vi "RudderToPoint.vi"(0 "Waypoint":T2 {"North" format="%#_10f"; "East" format="%#_8f"}, 1 "Robot Location":T2 {"North" format="%#_10f"; "East" format="%#_8f"}, 2 "Robot Heading":dbl, 3 "Angle to Check":dbl) -> (7 "Suggested Rudder Setpoint":T1 min=-1.0 max=1.0)   [LabVIEW 2012]
doc: "Takes in an angle to check, and returns a goodness value related to how close said angle is to the angle between the robot and the waypoint.\n\n**I find the above statement very unclear. What this vi should do now (perhaps this wasn't the original point, I can't tell) is take in the angle of the boat relative to the target, and use the rudder to point the boat at the target. This is done by putting a control loop around the boat-to-waypoint angle and making it go to zero. The control loop should be adjusted so that you get a more extreme reaction from the rudder at lower speeds. At a very low speed cutoff perhaps the rudder should just be set to 0, to save battery from the rudder twitching back and forth.**\n\nModified by Eric Schneider, Jan. 2014"
uses:
  Data/TypeDefs/UTM Location.ctl
  Data/TypeDefs/Rudder Set Suggestions.ctl
  Utilities/Math/Angles/Angle/Angle.lvclass
panel:
  out "Goodness":dbl
  # "TODO: Update the awful documentation"
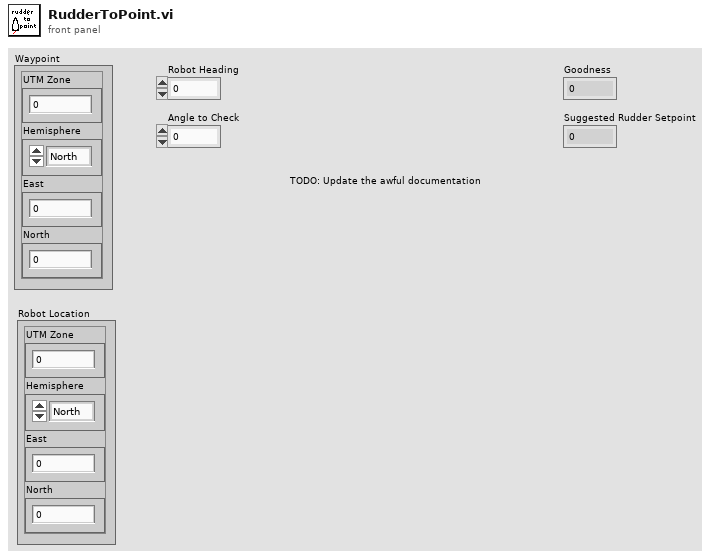
[diagram p1: front panel]
types:
  T1 = typedef "Rudder Set Suggestions.ctl" = dbl
  T2 = typedef "UTM Location.ctl" = cluster{"UTM Zone":dbl, "Hemisphere":enum16{"North", "South"}, "East":dbl, "North":dbl}
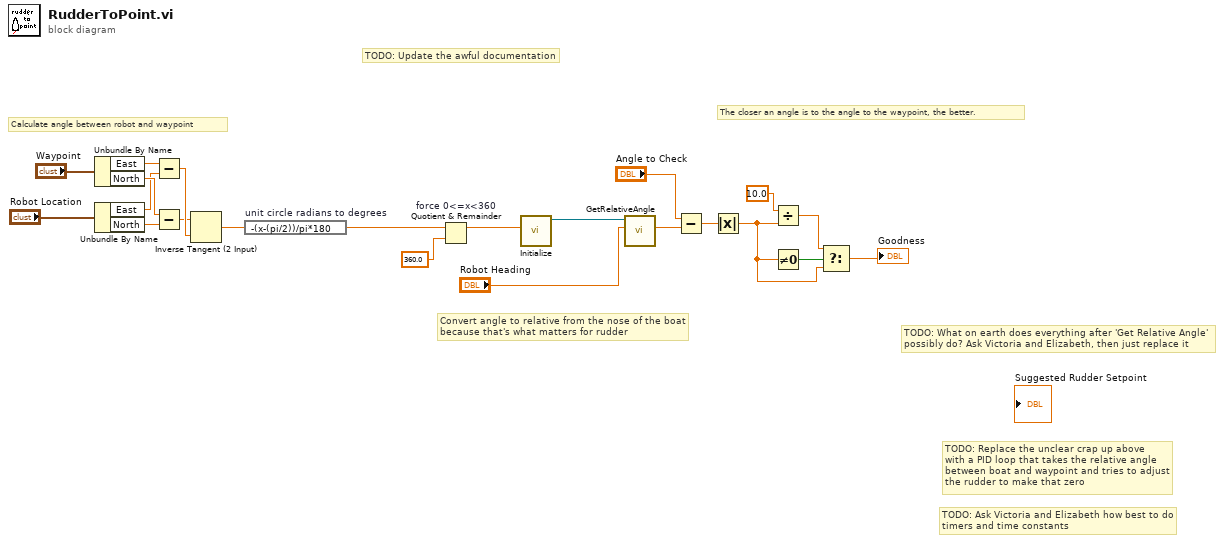
[diagram p0: block diagram]
diagram:
  # "TODO: Ask Victoria and Elizabeth how best to do\ntimers and time constants"
  # "TODO: Replace the unclear crap up above\nwith a PID loop that takes the relative angle\nbetween boat and waypoint and tries to adjust\nthe rudder to make that zero"
  # "TODO: What on earth does everything after 'Get Relative Angle'\npossibly do? Ask Victoria and Elizabeth, then just replace it"
  # "TODO: Update the awful documentation"
  # "The closer an angle is to the angle to the waypoint, the better."
  # "Convert angle to relative from the nose of the boat\nbecause that's what matters for rudder"
  # "Calculate angle between robot and waypoint"
  n1 = Unbundle By Name("Waypoint") -> ("East"=w17:dbl, "North"=w19:dbl)
  n2 = Unbundle By Name("Robot Location") -> ("East"=w18:dbl, "North"=w20:dbl)
  n3 = Subtract(x=w17, y=w18) -> (x-y=w22:dbl)
  n4 = Subtract(x=w19, y=w20) -> (x-y=w21:dbl)
  n5 = Inverse Tangent (2 Input) ("use inverse tangent\nto get heading")(1:w22, 2:w21) -> (0:w12:dbl)
  n6 = expression code="-(x-(pi/2))/pi*180" "unit circle radians to degrees"(w12) -> (w13:dbl)
  n7 = Quotient & Remainder "force 0<=x<360"(x=w13, y=360.0) -> (x-y*floor(x/y)=w11:dbl)  [unwired: 1 out]
  n8 = call "Initialize.vi"("Input Angle (Deg.)"=w11) -> ("Angle out"=w10:refnum<class "Angle.lvclass">)  [unwired: 9 in, 1 out]
  n9 = call "GetRelativeAngle.vi"("Boat Heading (Deg.)"="Robot Heading", "Angle in"=w10) -> ("Relative Angle"=w8:dbl)  [unwired: 8 in, 1 out]
  n10 = Subtract(x="Angle to Check", y=w8) -> (x-y=w6:dbl)
  n11 = Absolute Value(x=w6) -> (abs(x)=w2:dbl)
  n12 = Divide(x=10.0, y=w2) -> (x/y=w3:dbl)
  n13 = Not Equal To 0?(x=w2) -> (x != 0?=w4:bool)
  n14 = Select(t=w3, s=w4, f=w2) -> (s? t:f=→"Goodness":dbl)
